vi "4155C Config Sampling Measurements FPP v3.0.vi"(0 "VISA session":refnum<visa-resource-name>, 1 "Gate Compliance":dbl format="%.2f", 2 "FPP - Source":u32(ring)=6 items=["SMU1  ", "SMU2  ", "SMU3  ", "SMU4  ", "SMU5  ", "SMU6  ", "VSU1  ", "VSU2  "], 3 "FPP - Drain":u32(ring)=1 items=["SMU1  ", "SMU2  ", "SMU3  ", "SMU4  ", "SMU5  ", "SMU6  ", "VSU1  ", "VSU2  "], 4 "Drain Compliance":dbl format="%.2f", 5 "error in (no error)":errorcluster, 6 "Num Points":i16=1 min=1 max=1001, 7 "Timings":T2={"integration time"=0, "Short/Long integration time"=0.00064, "hold time (sec)"=0.0, "delay time (sec)"=0.0, "Step Time (0 disables)"=0.0, "sweep method"=0, "Pulse period"=0.005, "Base voltage"=0.0, "Pulse width"=0.0005} {"Pulse width" min=0.0005 max=0.1 step=0.0001 format="%.4f"; "Base voltage" min=-100.0 max=100.0 format="%^.4e"; "Pulse period" min=0.005 max=1.0 step=0.0001 format="%.4f"; "sweep method" items=["Continuous", "Pulsed"]; "Step Time (0 disables)" format="%.2f"; "delay time (sec)" min=0.0 format="%.4f"; "hold time (sec)" min=0.0 format="%.4f"; "Short/Long integration time" min=0.0 format="%^.0e"; "integration time" scale=0.0..2.0}, 8 "FPP - Gate":u32(ring)=2 items=["SMU1  ", "SMU2  ", "SMU3  ", "SMU4  ", "SMU5  ", "SMU6  ", "VSU1  ", "VSU2  "], 9 "FPP - Probe 1":u32(ring) items=["SMU1  ", "SMU2  ", "SMU3  ", "SMU4  ", "SMU5  ", "SMU6  ", "VSU1  ", "VSU2  "], 10 "Vg":dbl min=-100.0 max=100.0 format="%.2f", 11 "Vd":dbl min=-100.0 max=100.0 format="%.2f", 12 "Display on/off":bool, 13 "Sample time":dbl min=0.0 max=100000000000.0 format="%.2f", 15 "Sampling mode":u32(slide) scale=0.0..4.0, 16 "FPP - Probe 2":u32(ring)=3 items=["SMU1  ", "SMU2  ", "SMU3  ", "SMU4  ", "SMU5  ", "SMU6  ", "VSU1  ", "VSU2  "], 18 "Standby":T1) -> (14 "dup VISA resource name":refnum<visa-resource-name>, 19 "error out":errorcluster)   [LabVIEW 2016]
doc: "This VI configures the primary sweep source (VAR1) for a sweep mode measurement. \n* This VI does not perform error checking on MEASUREMENT MODE or UNIT TYPE of VAR1, therefore it is the application programmer's responsibility to make certain this VI is used in the proper mode."
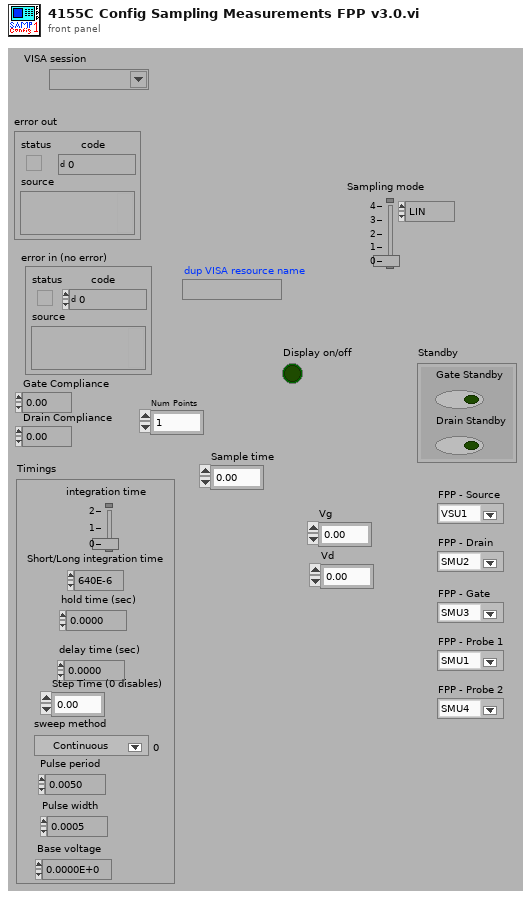
[diagram p1: front panel]
types:
  T1 = cluster{"Gate Standby":bool, "Drain Standby":bool}
  T2 = cluster{"integration time":u32, "Short/Long integration time":dbl, "hold time (sec)":dbl, "delay time (sec)":dbl, "Step Time (0 disables)":dbl, "sweep method":u16, "Pulse period":dbl, "Base voltage":dbl, "Pulse width":dbl}
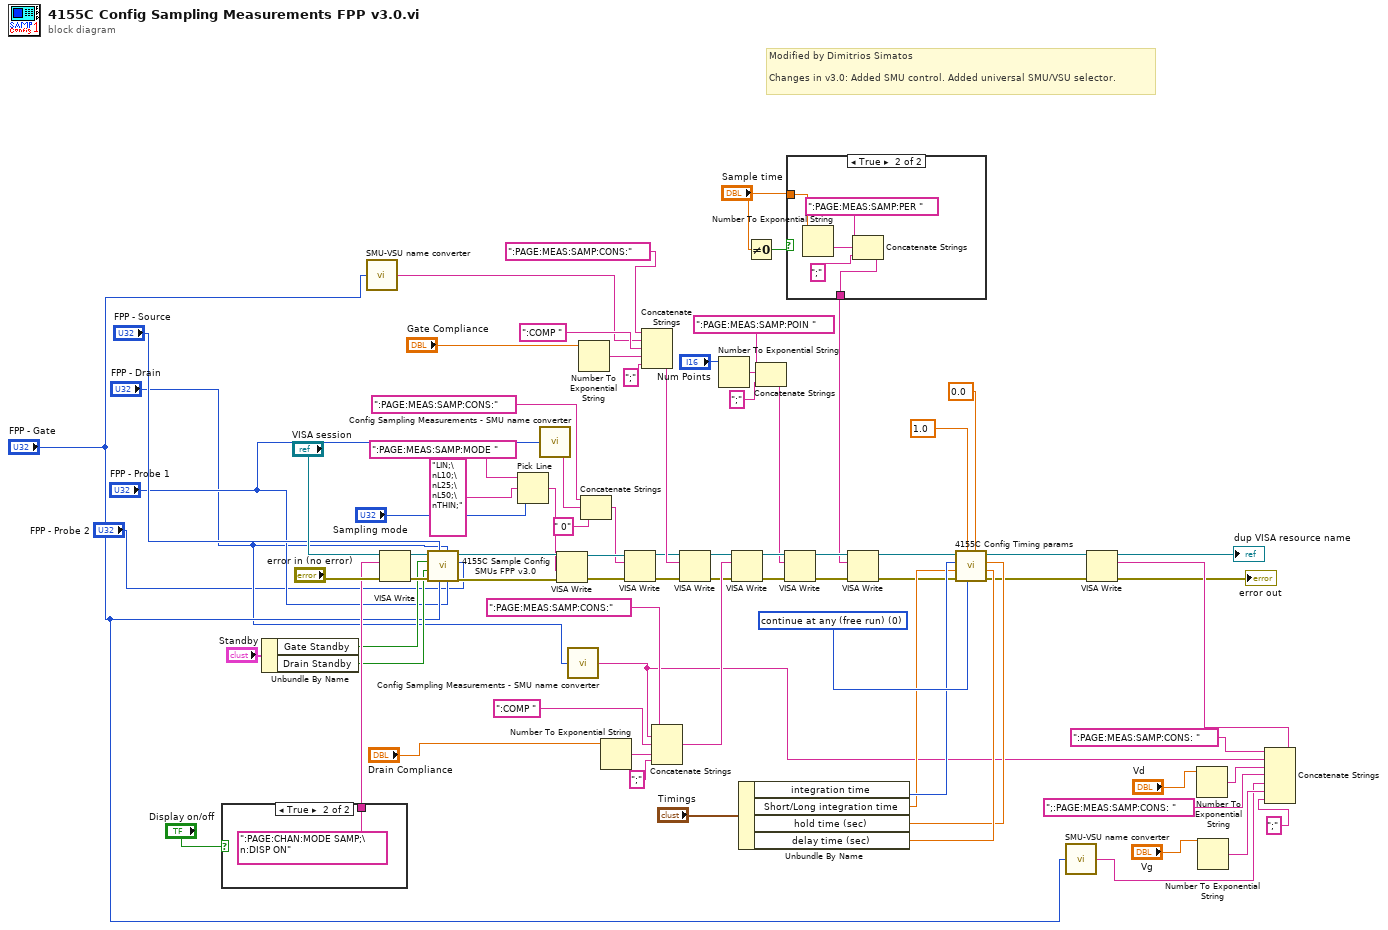
[diagram p0: block diagram]
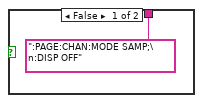
[diagram p2: hidden frame]
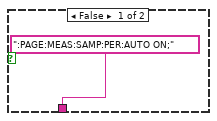
[diagram p3: hidden frame]
diagram:
  w65 = u8 0 items=["continue at any (free run)", "stop at any abnorm", "stop at compliance"] ("stop condition (free run:0)")
  # "Modified by Dimitrios Simatos\n\nChanges in v3.0: Added SMU control. Added universal SMU/VSU selector."
  n1 = case shown="True" "Display on/off" {
    tunnel: [":PAGE:CHAN:MODE SAMP;\n:DISP OFF" ("write buffer (\"\")") ":PAGE:CHAN:MODE SAMP;\n:DISP ON" ("write buffer (\"\")")] -> w38
    frame False {
    }
    frame True {
    }
  }
  n2 = Unbundle By Name("Standby") -> ("Gate Standby"=w28:bool, "Drain Standby"=w27:bool)
  n3 = call "SMU-VSU name converter.vi"("unit to configure"="FPP - Gate") -> ("SMU/VSU to be configured"=w16:string)
  n4 = VISA Write(VISA resource name="VISA session", write buffer=w38, error in (no error)="error in (no error)") -> (VISA resource name out=w56:refnum<visa-resource-name>, error out=w55:errorcluster)  [unwired: 1 out]
  n5 = call "4155C Sample Config SMUs FPP v3.0.vi"("FPP - Probe 2"="FPP - Probe 2", "FPP - Probe 1"="FPP - Probe 1", "FPP - Drain"="FPP - Drain", "FPP - Gate"="FPP - Gate", "FPP - Source"="FPP - Source", "error in (no error)"=w55, "Drain Standby"=w27, "Gate Standby"=w28, "VISA resource name in"=w56) -> ("error out"=w35:errorcluster, "VISA Resource Name out"=w34:refnum<visa-resource-name>)  [unwired: 1 in]
  n6 = Pick Line(string ("")=":PAGE:MEAS:SAMP:MODE ", multi-line string="LIN;\nL10;\nL25;\nL50;\nTHIN;", line index="Sampling mode") -> (output string=w30:string)
  n7 = call "Config Sampling Measurements - SMU name converter.vi"("unit to configure"="FPP - Probe 1") -> ("SMU to be configured"=w13:string)
  n8 = VISA Write(VISA resource name=w34, write buffer=w30, error in (no error)=w35) -> (VISA resource name out=w37:refnum<visa-resource-name>, error out=w36:errorcluster)  [unwired: 1 out]
  n9 = call "Config Sampling Measurements - SMU name converter.vi"("unit to configure"="FPP - Drain") -> ("SMU to be configured"=w9:string)
  n10 = Number To Exponential String(number="Gate Compliance") -> (E-format string=w72:string)  [unwired: 3 in]
  n11 = Concatenate Strings(":PAGE:MEAS:SAMP:CONS:" ("write buffer (\"\")"), w13, " 0" ("write buffer (\"\")")) -> (w15:string)
  n12 = Number To Exponential String(number="Drain Compliance") -> (E-format string=w74:string)  [unwired: 3 in]
  n13 = VISA Write(VISA resource name=w37, write buffer=w15, error in (no error)=w36) -> (VISA resource name out=w70:refnum<visa-resource-name>, error out=w69:errorcluster)  [unwired: 1 out]
  n14 = Concatenate Strings(":PAGE:MEAS:SAMP:CONS:", w16, ":COMP ", w72, ";" ("Substring")) -> (w73:string)
  n15 = Concatenate Strings(":PAGE:MEAS:SAMP:CONS:", w9, ":COMP ", w74, ";" ("Substring")) -> (w77:string)
  n16 = VISA Write(VISA resource name=w70, write buffer=w73, error in (no error)=w69) -> (VISA resource name out=w68:refnum<visa-resource-name>, error out=w67:errorcluster)  [unwired: 1 out]
  n17 = Number To Exponential String(number="Num Points") -> (E-format string=w53:string)  [unwired: 3 in]
  n18 = VISA Write(VISA resource name=w68, write buffer=w77, error in (no error)=w67) -> (VISA resource name out=w78:refnum<visa-resource-name>, error out=w79:errorcluster)  [unwired: 1 out]
  n19 = Unbundle By Name("Timings") -> ("integration time"=w62:u32, "Short/Long integration time"=w59:dbl, "hold time (sec)"=w63:dbl, "delay time (sec)"=w64:dbl)
  n20 = Not Equal To 0?(x="Sample time") -> (x != 0?=w45:bool)
  n21 = Concatenate Strings(":PAGE:MEAS:SAMP:POIN " ("write buffer (\"\")"), w53, ";" ("Substring")) -> (w47:string)
  n22 = VISA Write(VISA resource name=w78, write buffer=w47, error in (no error)=w79) -> (VISA resource name out=w44:refnum<visa-resource-name>, error out=w43:errorcluster)  [unwired: 1 out]
  n23 = case shown="True" w45 {
    tunnel: "Sample time" -> [_ w86]
    tunnel: [":PAGE:MEAS:SAMP:PER:AUTO ON;" w83] -> w40
    frame False {
    }
    frame True {
      n24 = Number To Exponential String(number=w86) -> (E-format string=w87:string)  [unwired: 3 in]
      n25 = Concatenate Strings(":PAGE:MEAS:SAMP:PER " ("Substring"), w87, ";" ("Substring")) -> (w83:string)
    }
  }
  n26 = VISA Write(VISA resource name=w44, write buffer=w40, error in (no error)=w43) -> (VISA resource name out=w41:refnum<visa-resource-name>, error out=w42:errorcluster)  [unwired: 1 out]
  n27 = call "4155C Config Timing params.vi"("delay time (sec)"=w64, "hold time (sec)"=w63, "Step Time (0 disables)"=0.0, "stop condition (free run:0)"=w65, "wait time parameter"=1.0, "error in (no error)"=w42, "Short/Long integration time"=w59, "integration time"=w62, "VISA session"=w41) -> ("error out"=w20:errorcluster, "dup VISA resource name"=w21:refnum<visa-resource-name>)  [unwired: 1 in]
  n28 = call "SMU-VSU name converter.vi"("unit to configure"="FPP - Gate") -> ("SMU/VSU to be configured"=w6:string)
  n29 = Number To Exponential String(number="Vd") -> (E-format string=w25:string)  [unwired: 3 in]
  n30 = Number To Exponential String(number="Vg") -> (E-format string=w7:string)  [unwired: 3 in]
  n31 = Concatenate Strings(":PAGE:MEAS:SAMP:CONS: " ("write buffer (\"\")"), w9, w25, ";:PAGE:MEAS:SAMP:CONS: " ("write buffer (\"\")"), w6, w7, ";" ("Substring")) -> (w22:string)
  n32 = VISA Write(VISA resource name=w21, write buffer=w22, error in (no error)=w20) -> (VISA resource name out=→"dup VISA resource name":refnum<visa-resource-name>, error out=→"error out":errorcluster)  [unwired: 1 out]
